vi "read fixed channel configuration.vi"(8 "error in":errorcluster, 11 "fixed channel editor node in":refnum<class "fixed channel editor.lvclass">) -> (0 "error out":errorcluster, 2 "fixed channel configuration":refnum<class "fixed channel configuration.lvclass">, 3 "fixed channel editor node out":refnum<class "fixed channel editor.lvclass">)   [LabVIEW 2013, in "fixed channel editor.lvclass"]
uses:
  fixed channel editor.lvclass
  module/configuration/fixed channel configuration.lvclass
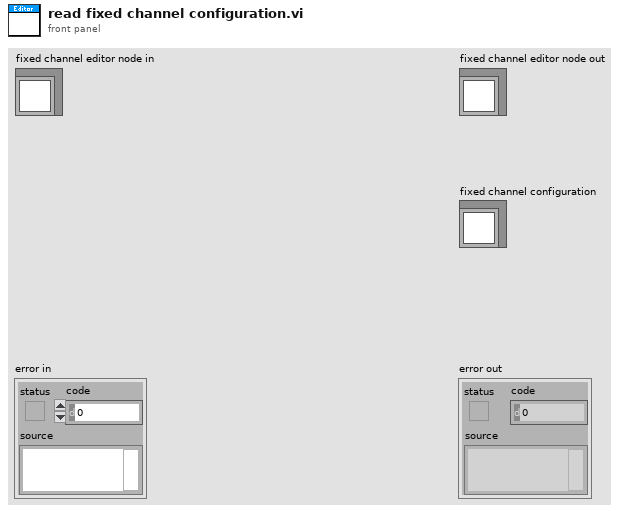
[diagram p1: front panel]
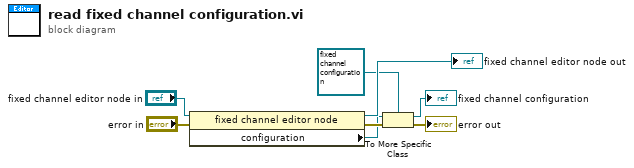
[diagram p0: block diagram]
diagram:
  n1 = property class="fixed channel editor node"(reference="fixed channel editor node in", error in="error in") -> (reference out=→"fixed channel editor node out":refnum<class "fixed channel editor.lvclass">, error out=w7:errorcluster, "configuration"=w3:refnum<class "NISE_CEF_serializable configuration.lvclass">)
  n2 = To More Specific Class(target class=refnum<class "fixed channel configuration.lvclass"> refnum ("fixed channel configuration"), reference=w3, error in=w7) -> (specific class reference=→"fixed channel configuration":refnum<class "fixed channel configuration.lvclass">, error out=→"error out":errorcluster)
